vi "Launch Async Handler.vi"(8 "error in (no error)":errorcluster, 9 "Message Data":variant, 10 "Message":string, 11 "Async Action In":refnum<class "Async Handler.lvclass">) -> (0 "error out":errorcluster, 3 "Async Action Out":refnum<class "Async Handler.lvclass">)   [LabVIEW 2020, in "Async Handler.lvclass"]
doc: "Launches an asynchronous helper loop. Multiple helper loops may be launched using multiple calls to this VI. The Message and Message Data provided to this VI will be available in the Helper Action.vi once running."
uses:
  Async Handler.lvclass
  Private/Async Handler.vi
  Process/Process.lvclass
  <vilib>/Utility/error.llb/Error Cluster From Error Code.vi
  <vilib>/ErrorRing/Error Ring.xnode
  Process/Public/Lifecycle/API Mode.ctl
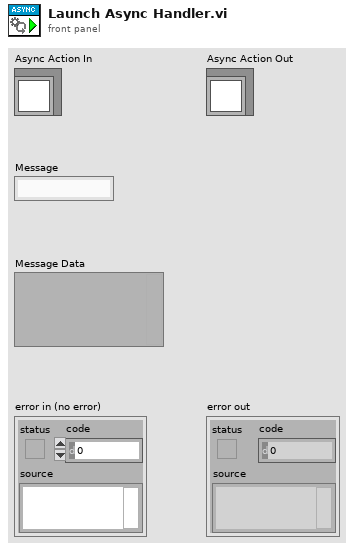
[diagram p1: front panel]
types:
  T1 = typedef "Process.lvclass/API Mode.ctl" = enum16{"Send Message", "Handle Message"}
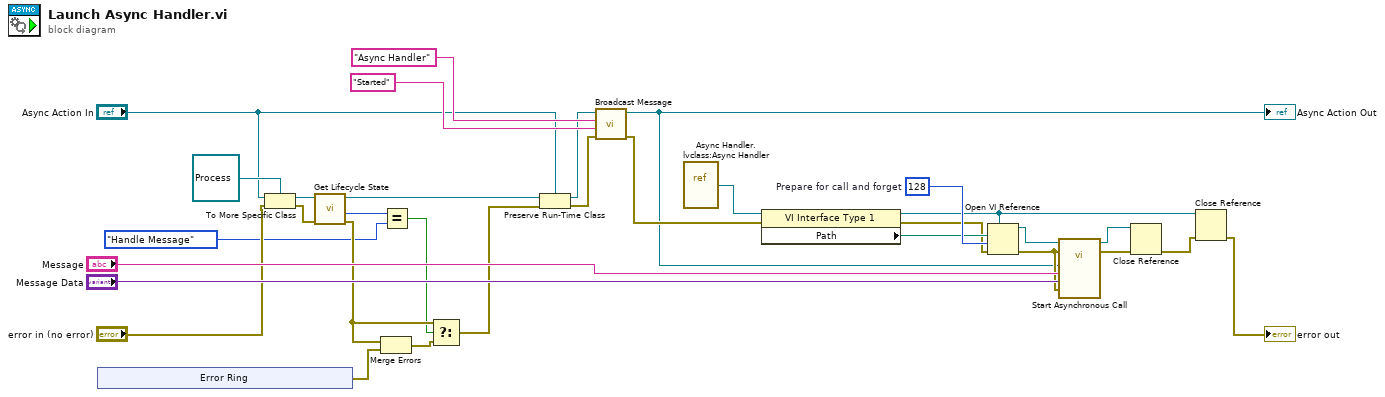
[diagram p0: block diagram]
diagram:
  w26 = 128  # Prepare for call and forget
  n1 = xnode "Error Ring"() -> ("error out"=w14:errorcluster)
  n2 = To More Specific Class(target class=refnum<class "Process.lvclass"> refnum ("Process Out"), reference="Async Action In", error in="error in (no error)") -> (specific class reference=w19:refnum<class "Process.lvclass">, error out=w18:errorcluster)
  n3 = call "Get Lifecycle State.vi"("error in (no error)"=w18, "Process In"=w19) -> ("error out"=w17:errorcluster, "API Mode"=w16:T1, "Process Out"=w7:refnum<class "Process.lvclass">)  [unwired: 6 in, 1 out]
  n4 = Merge Errors(w17, w14) -> (w15:errorcluster)
  n5 = Equal?(x=w16, y=API_Mode."Handle Message") -> (x = y?=w2:bool)
  n6 = Select(t=w17, s=w2, f=w15) -> (s? t:f=w6:errorcluster)
  n7 = Preserve Run-Time Class(object in=w7, error in=w6, 2:"Async Action In") -> (object out=w3:refnum<class "Async Handler.lvclass">, error out=w5:errorcluster)
  n8 = call-dynamic "Broadcast Message.vi"("error in (no error)"=w5, "Message Data"="Started", "Message"="Async Handler", "Asynchronous Action In"=w3) -> ("error out"=w10:errorcluster, "Asynchronous Action Out"=w9:refnum<class "Async Handler.lvclass">)  [unwired: 6 in]
  "Async Action Out" <- w9
  n9 = vi-ref "Async Handler.lvclass:Async Handler.vi"() -> (w27:refnum<vi>)
  n10 = property class="VI Interface Type 1"(reference=w27, error in=w10) -> (reference out=w20:refnum<vi>, error out=w22:errorcluster, "Path"=w24:path)
  n11 = Open VI Reference(type specifier VI Refnum (for type only)=w20, vi path=w24, options=w26, error in (no error)=w22) -> (vi reference=w25:refnum<vi>, error out=w23:errorcluster)  [unwired: 2 in]
  n12 = call-by-ref "Start Asynchronous Call"(reference=w25, error in=w23, 8:"error in (no error)"=w23, "Message Data"="Message Data", "Message"="Message", "Asynchronous Action In"=w9) -> (reference out=w29:refnum<vi>, error out=w28:errorcluster)  [unwired: 6 in, 2 out]
  n13 = Close Reference(reference=w29, error in (no error)=w28) -> (error out=w21:errorcluster)
  n14 = Close Reference(reference=w20, error in (no error)=w21) -> (error out=→"error out":errorcluster)
